vi "read typedef clusters for channel info.vi"(11 "fixed channel configuration":refnum<class "fixed channel configuration.lvclass">) -> (0 "error out":errorcluster, 1 "Channel Counts":i32[](array[numeric]), 2 "> Categorized name list >":string[][](array[string]), 3 "> Uncategorized name list >":string[](array[string]))   [LabVIEW 2013, in "fixed channel configuration.lvclass"]
uses:
  fixed channel configuration.lvclass
  <vilib>/NI/Tag Bus Module Framework/channel/TBM channel.lvclass
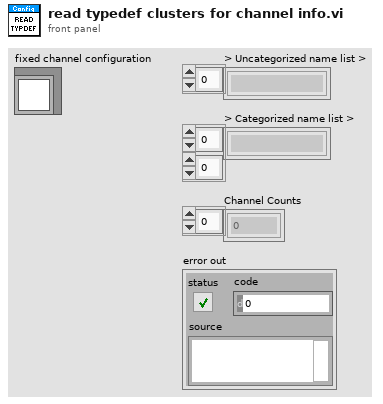
[diagram p1: front panel]
types:
  T1 = typedef "TBM channel.lvclass/channel classification.ctl" = enum16{"input data", "output data", "processing parameter", "processing result"}
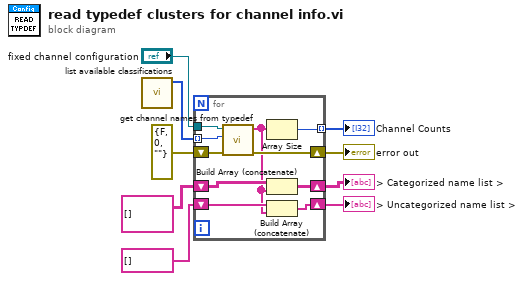
[diagram p0: block diagram]
diagram:
  n1 = call <vilib>:"list available classifications.vi"() -> ("supported types"=w1:T1[])  [unwired: 11 in]
  n2 = for {
    tunnel: w1 -> [w11] mode=indexing
    shift-right: [w19] -> w6
    shift-left: string[][] [] -> [w18]
    shift-right: [w17] -> w9
    shift-left: errorcluster {"status"=FALSE, "code"=0, "source"=""} ("error out") -> [w16]
    shift-right: [w15] -> w8
    shift-left: string[] [] -> [w14]
    tunnel: [w12] -> w3 mode=indexing
    tunnel: "fixed channel configuration" -> [w10]
    n3 = call "get channel names from typedef.vi"("error in"=w16, "channel classification"=w11, "fixed channel configuration"=w10) -> ("error out"=w17:errorcluster, "Channel Names"=w13:string[])  [unwired: 7 in]
    n4 = Array Size(array=w13) -> (size(s)=w12:i32)
    n5 = Build Array (concatenate)(w18, w13) -> (w19:string[][])
    n6 = Build Array (concatenate)(w14, w13) -> (w15:string[])
  }
  "error out" <- w9
  "> Uncategorized name list >" <- w8
  "> Categorized name list >" <- w6
  "Channel Counts" <- w3
